vi "dataset.create_begin.vi"(8 "error in":errorcluster, 10 "name":string, 11 "Client in":refnum<class "Client.lvclass">) -> (0 "error out":errorcluster, 2 "DatasetCreateStaging":refnum<class "DatasetCreateStaging.lvclass">, 3 "Client out":refnum<class "Client.lvclass">)   [LabVIEW 2020, in "Client.lvclass"]
doc: "Creates a new empty dataset with the given name and optional description and returns a handle to it."
uses:
  Client.lvclass
  Client.lvclass/Client.ctl
  client.lvlib
  DatasetCreateStaging/DatasetCreateStaging.lvclass
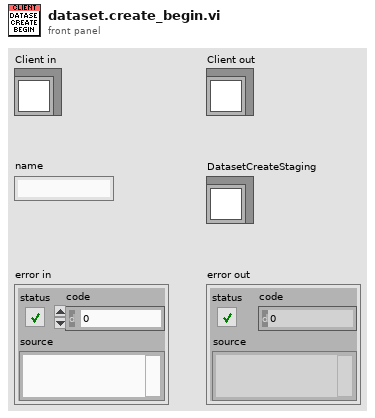
[diagram p1: front panel]
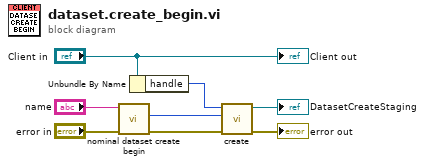
[diagram p0: block diagram]
diagram:
  n1 = call "nominal dataset create begin.vi"("error in (no error)"="error in", "name"="name") -> ("error out"=w3:errorcluster, "out_staging out"=w4:i32)  [unwired: 7 in, 1 out]
  n2 = Unbundle By Name("Client in") -> ("handle"=w5:i32)
  n3 = call "create.vi"("error in (no error)"=w3, "handle"=w4, "client"=w5) -> ("error out"=→"error out":errorcluster, "DatasetCreateStaging"=→"DatasetCreateStaging":refnum<class "DatasetCreateStaging.lvclass">)  [unwired: 7 in]
  "Client out" <- "Client in"
